vi "StepperMotorPWM (SubVI).vi"(4 "Reset":bool, 6 "steps/rev":dbl=6400.0 format="%#_13g", 7 "EN [L,R]":bool, 8 "error in (no error)":errorcluster, 9 "LoopTime":dbl=0.005 format="%#_13g", 10 "Speed (deg/s) [L,R]":dbl[](array[numeric])=[0.0, 0.0]) -> (0 "error out (no error)":errorcluster, 2 "DegreeCounter":dbl[](array[numeric]))   [LabVIEW 2019]
uses:
  <vilib>/myRIO/Instrument Drivers/Onboard IO/DIO/typedefs/DIO Reference.ctl
  <vilib>/myRIO/Common/Instrument Driver Framework/Utilities/typedefs/myRIO Generic Hardware Reference.ctl
  <vilib>/myRIO/Common/Instrument Driver Framework/Utilities/typedefs/Hardware Version Enum.ctl
  <vilib>/myRIO/Common/Instrument Driver Framework/Utilities/typedefs/myRIO v1.0 Reference.ctl
  <vilib>/myRIO/Common/Instrument Driver Framework/Utilities/typedefs/Generic FPGA Reference.ctl
  <vilib>/myRIO/Common/Instrument Driver Framework/myRIO v1.0/DIO/typedefs/DIO Channels List.ctl
  <vilib>/myRIO/Common/Instrument Driver Framework/myRIO v1.0/DIO/typedefs/DIO Channels Enum.ctl
  <vilib>/userDefined/High Color/nirio_resource_hc.ctl
  <vilib>/myRIO/Instrument Drivers/Onboard IO/PWM/typedefs/PWM Reference.ctl
  <vilib>/myRIO/Common/Instrument Driver Framework/myRIO v1.0/PWM/typedefs/PWM Channels Enum.ctl
  <vilib>/myRIO/Instrument Drivers/Onboard IO/PWM/typedefs/PWM Configuration.ctl
  <vilib>/myRIO/Common/Instrument Driver Framework/Utilities/vis/Is FPGA Ref Available.vi
  <vilib>/myRIO/Common/Instrument Driver Framework/myRIO v1.0/DIO/vis/myRIO v1.1 Open DIO.vi
  <vilib>/myRIO/Instrument Drivers/Onboard IO/DIO/vis/Write.vi
  <vilib>/myRIO/Common/Instrument Driver Framework/myRIO v1.0/PWM/vis/myRIO v1.1 Open PWM.vi
  <vilib>/myRIO/Instrument Drivers/Onboard IO/PWM/vis/Set Duty Cycle and Frequency.vi
  <vilib>/myRIO/Common/Instrument Driver Framework/Utilities/vis/Validate Channels.vi
  <vilib>/myRIO/Common/Instrument Driver Framework/myRIO v1.0/DIO/vis/myRIO v1.0 Reserve DIO.vi
  <vilib>/myRIO/Common/Instrument Driver Framework/myRIO v1.0/PWM/vis/myRIO v1.0 Reserve PWM.vi
  <vilib>/myRIO/Common/Instrument Driver Framework/myRIO v1.0/Resource Manager/vis/myRIO v1.0 Reserve Channel List.vi
  <vilib>/myRIO/Common/Instrument Driver Framework/myRIO v1.0/DIO/vis/myRIO v1.0 Build MUX Configuration DIO.vi
  <vilib>/myRIO/Common/Instrument Driver Framework/myRIO v1.0/PWM/vis/myRIO v1.0 Build MUX Configuration PWM.vi
  <vilib>/myRIO/Common/Instrument Driver Framework/myRIO v1.0/Resource Manager/vis/myRIO v1.0 Reserve Channel.vi
  <vilib>/myRIO/Common/Instrument Driver Framework/myRIO v1.0/Resource Manager/vis/myRIO v1.0 Unreserve Channel.vi
  <vilib>/myRIO/Common/Instrument Driver Framework/myRIO v1.0/Resource Manager/vis/myRIO v1.0 Create Configuration List.vi
  <vilib>/myRIO/Common/Instrument Driver Framework/myRIO v1.0/Resource Manager/vis/myRIO v1.0 Build Mutex Name.vi
  <vilib>/Utility/VariantDataType/GetNumericInfo.vi
  <vilib>/Utility/error.llb/Error Cluster From Error Code.vi
  <vilib>/myRIO/Common/Instrument Driver Framework/myRIO v1.0/myRIO v1.1 Open.vi
  <vilib>/myRIO/Common/Instrument Driver Framework/Utilities/vis/IO Manager.vi
  <vilib>/myRIO/Common/Instrument Driver Framework/Utilities/vis/Configuration Manager.vi
  <vilib>/myRIO/Common/Instrument Driver Framework/myRIO v1.0/Resource Manager/vis/myRIO v1.0 Configure IO.vi
  <vilib>/myRIO/Common/Instrument Driver Framework/myRIO v1.0/myRIO v1.0 Close.vi
  <vilib>/myRIO/Common/Instrument Driver Framework/myRIO v1.0/DIO/vis/myRIO v1.0 Write DIO.vi
  <vilib>/myRIO/Common/Instrument Driver Framework/myRIO v1.0/PWM/vis/myRIO v1.0 Write PWM.vi
  <vilib>/myRIO/Express VI/Onboard IO/DO/DO Express VI.xnode
  <vilib>/myRIO/Instrument Drivers/Onboard IO/DIO/vis/myRIO DIO Open.xnode
  <vilib>/myRIO/Express VI/Onboard IO/PWM/PWM Express VI.xnode
  <vilib>/myRIO/Instrument Drivers/Onboard IO/PWM/vis/myRIO PWM Open.xnode
  <vilib>/myRIO/Instrument Drivers/Onboard IO/PWM/PWM.lvlib
  <vilib>/myRIO/Instrument Drivers/Onboard IO/DIO/DIO.lvlib
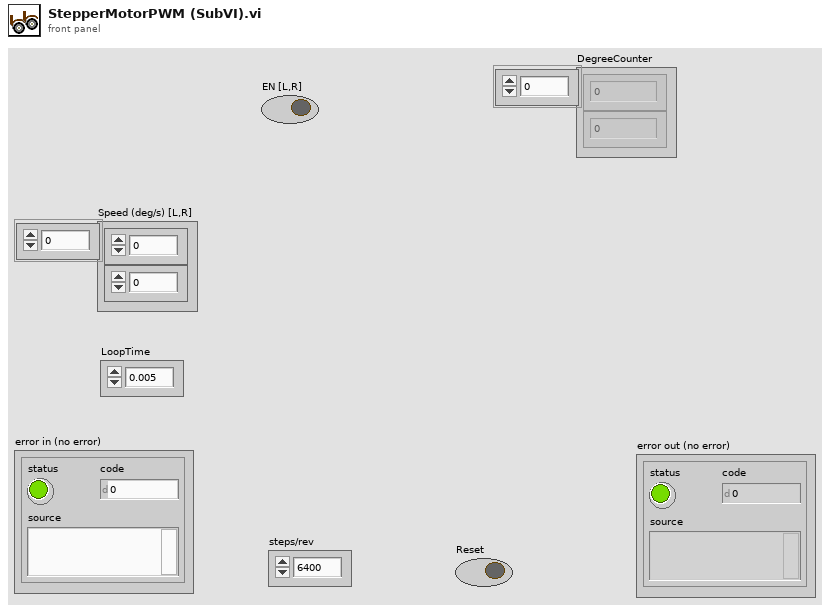
[diagram p1: front panel]
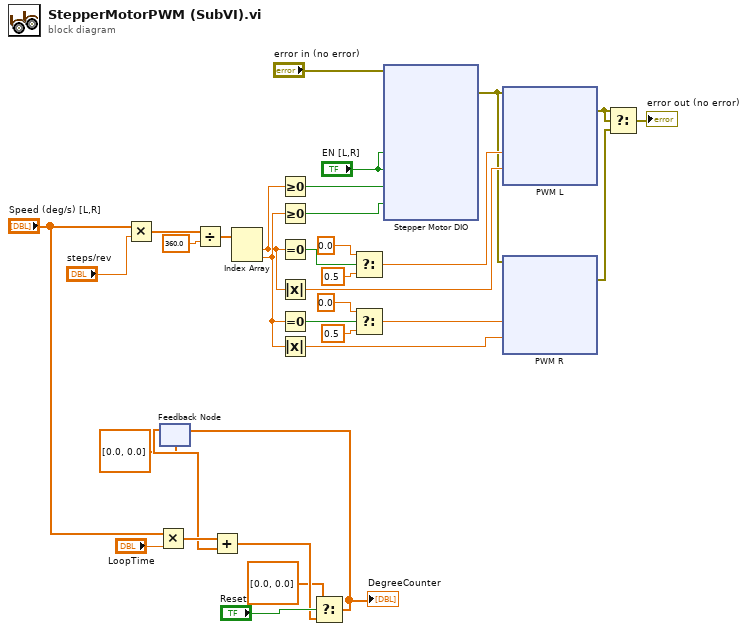
[diagram p0: block diagram]
diagram:
  n1 = Multiply(x="Speed (deg/s) [L,R]", y="steps/rev") -> (x*y=w14:dbl[])
  n2 = Multiply(x="Speed (deg/s) [L,R]", y="LoopTime") -> (x*y=w7:dbl[])
  n3 = feedback #1(dbl[] [0.0, 0.0]) -> (w6:dbl[])
  n4 = Divide(x=w14, y=360.0) -> (x/y=w11:dbl[])
  n5 = Add(x=w7, y=w6) -> (x+y=w2:dbl[])
  n6 = Index Array(array=w11) -> (element #1=w28:dbl, element #2=w30:dbl)  [unwired: 2 in]
  n7 = Greater Or Equal To 0?(x=w28) -> (x >= 0?=w29:bool)
  n8 = Greater Or Equal To 0?(x=w30) -> (x >= 0?=w31:bool)
  n9 = Equal To 0?(x=w28) -> (x = 0?=w20:bool)
  n10 = Absolute Value(x=w28) -> (abs(x)=w33:dbl)
  n11 = Equal To 0?(x=w30) -> (x = 0?=w26:bool)
  n12 = Absolute Value(x=w30) -> (abs(x)=w32:dbl)
  n13 = Select(t=dbl[] [0.0, 0.0], s="Reset", f=w2) -> (s? t:f=w3:dbl[])
  "DegreeCounter" <- w3
  n14 = feedback-in #1(w3) -> ()
  n15 = Select(t=0.0, s=w20, f=0.5) -> (s? t:f=w23:dbl)
  n16 = Select(t=0.0, s=w26, f=0.5) -> (s? t:f=w27:dbl)
  n17 = xnode "Stepper Motor DIO"("EN_L (A/DIO0 (Pin 11))"="EN [L,R]", "EN_R (A/DIO2 (Pin 15))"="EN [L,R]", "DIR_L (A/DIO1 (Pin 13))"=w29, "DIR_R (A/DIO3 (Pin 17))"=w31, "error in (no error)"="error in (no error)") -> ("error out"=w19:errorcluster)
  n18 = xnode "PWM L"("Duty Cycle"=w23, "Frequency [Hz]"=w33, "error in (no error)"=w19) -> ("error out"=w17:errorcluster)
  n19 = xnode "PWM R"("Duty Cycle"=w27, "Frequency [Hz]"=w32, "error in (no error)"=w19) -> ("error out"=w16:errorcluster)
  n20 = Select(t=w17, s=w17, f=w16) -> (s? t:f=→"error out (no error)":errorcluster)
